vi "RD_WR_init.vi"(0 "MVIName def":string[](array[string]), 1 "N_moduls":i32, 2 "Status Reference":T2, 3 "KFM":string[](array[string]), 5 "IP addr def":T4(array[cluster]), 7 "timeouts def":T3[](array[typedef]), 9 "start_stop def":bool[](array[boolean]), 11 "error in":errorcluster, 12 "WR en def":bool[](array[boolean]), 13 "conninfo system DB":T1, 14 "KFMTable":string="kfm_3") -> (4 "RD_WR param":T5, 15 "error":errorcluster)   [LabVIEW 2019, in "ICPCON_Param.lvlib"]
uses:
  ICPCON_Param.lvlib
  ICPCON Param.ctl
  Eth timeouts.ctl
  Eth Status/Ctl/Status.ctl
  MB_TCP2/MB_TCP_State.ctl
  Database/ctl/Coninfo.ctl
  Eth Status/Eth Status.lvlib
  Database/PostgreSQL.lvlib
  MB_TCP2/MB_TCP.lvclass
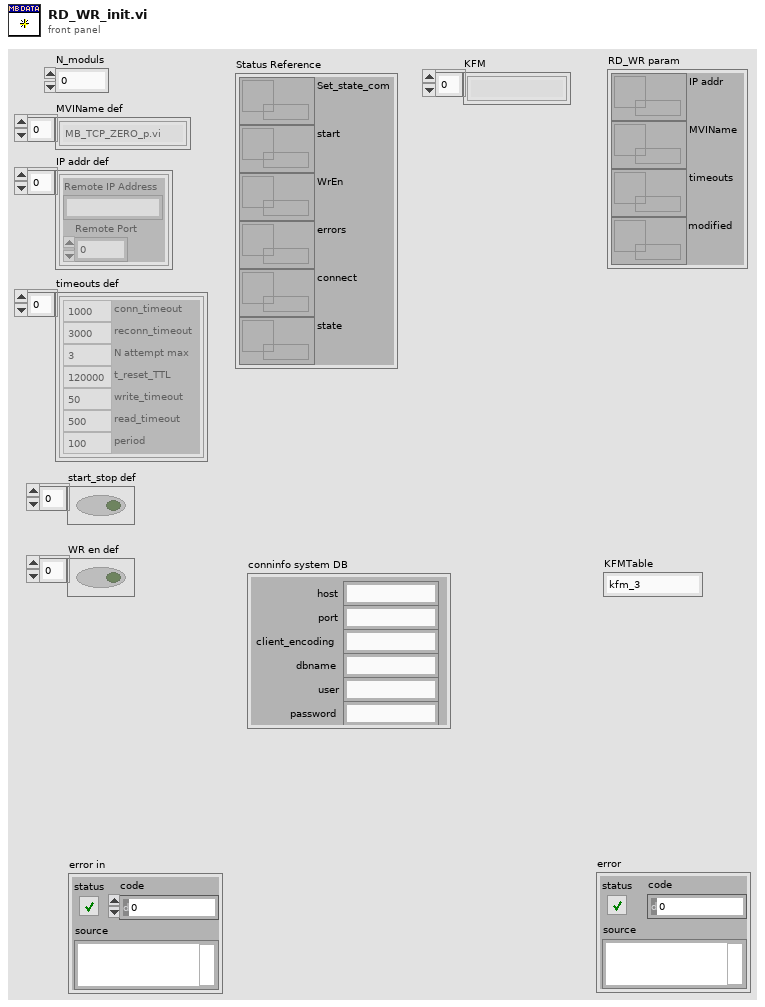
[diagram p1: front panel]
types:
  T1 = typedef "PostgreSQL.lvlib/Coninfo.ctl" = cluster{"host":string, "port":string, "client_encoding":string, "dbname":string, "user":string, "password":string}
  T2 = typedef "Eth Status.lvlib/Status.ctl" = cluster{"Set_state_com":refnum<data-value>, "start":refnum<data-value>, "WrEn":refnum<data-value>, "errors":refnum<data-value>, "connect":refnum<data-value>, "state":refnum<data-value>}
  T3 = typedef "ICPCON_Param.lvlib/Eth timeouts.ctl" = cluster{"conn_timeout":i32, "reconn_timeout":i32, "N attempt max":i32, "t_reset_TTL":i32, "write_timeout":i32, "read_timeout":i32, "period":i32}
  T4 = cluster{"Remote IP Address":string, "Remote Port":u16}[]
  T5 = typedef "ICPCON_Param.lvlib/ICPCON Param.ctl" = cluster{"IP addr":refnum<data-value>, "MVIName":refnum<data-value>, "timeouts":refnum<data-value>, "modified":refnum<data-value>}
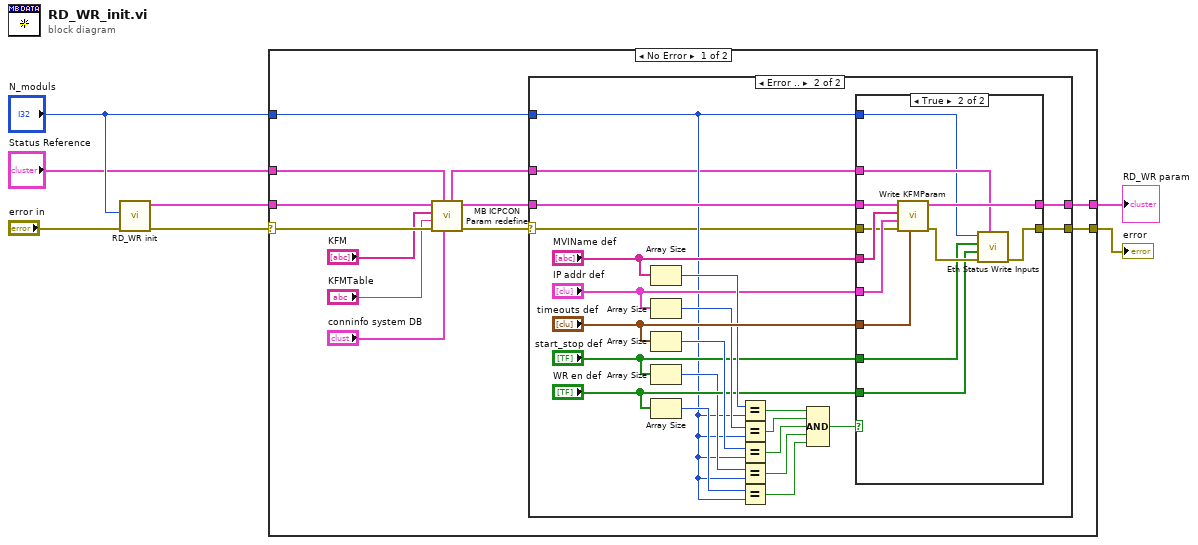
[diagram p0: block diagram]
diagram:
  n1 = call "RD_WR init.vi"("error in"="error in", "N_moduls"="N_moduls") -> ("error"=w2:errorcluster, "RD_WR param"=w5:T5)  [unwired: 8 in]
  n2 = case shown="No Error" w2 {
    selector: w2 -> [w14 w58]
    tunnel: [w18 w58] -> w3
    tunnel: w5 -> [w16 w59]
    tunnel: [w19 w59] -> w6
    tunnel: "N_moduls" -> [w15 _]
    tunnel: "Status Reference" -> [w13 _]
    frame No Error {
      n3 = call "MB ICPCON Param redefine.vi"("conninfo"="conninfo system DB", "Status Reference"=w13, "error in (no error)"=w14, "KFMTable"="KFMTable", "KFM param"="KFM", "KFM param in"=w16) -> ("error"=w11:errorcluster, "KFM param out"=w17:T5, "Status Reference out"=w12:T2)  [unwired: 3 in]
      n4 = case shown="Error .." w11 {
        selector: w11 -> [w20 w22]
        tunnel: [w20 w23] -> w18
        tunnel: w17 -> [w21 w43]
        tunnel: [w21 w25] -> w19
        tunnel: w15 -> [_ w26]
        tunnel: w12 -> [_ w24]
        frame No Error {
        }
        frame Error {
          n5 = Array Size(array="MVIName def") -> (size(s)=w39:i32)
          n6 = Array Size(array="IP addr def") -> (size(s)=w38:i32)
          n7 = Array Size(array="timeouts def") -> (size(s)=w37:i32)
          n8 = Array Size(array="start_stop def") -> (size(s)=w34:i32)
          n9 = Array Size(array="WR en def") -> (size(s)=w33:i32)
          n10 = Equal?(x=w39, y=w26) -> (x = y?=w40:bool)
          n11 = Equal?(x=w38, y=w26) -> (x = y?=w41:bool)
          n12 = Equal?(x=w37, y=w26) -> (x = y?=w32:bool)
          n13 = Equal?(x=w34, y=w26) -> (x = y?=w31:bool)
          n14 = Equal?(x=w33, y=w26) -> (x = y?=w30:bool)
          n15 = Compound Arithmetic op=AND(w40, w41, w32, w31, w30) -> (w29:bool)
          n16 = case shown="True" w29 {
            tunnel: "MVIName def" -> [_ w49]
            tunnel: "IP addr def" -> [_ w48]
            tunnel: [w44 w53] -> w23
            tunnel: w43 -> [w45 w57]
            tunnel: [w45 w56] -> w25
            tunnel: "timeouts def" -> [_ w55]
            tunnel: w24 -> [_ w52]
            tunnel: "start_stop def" -> [_ w51]
            tunnel: "WR en def" -> [_ w50]
            tunnel: w26 -> [_ w47]
            tunnel: w22 -> [w44 w46]
            frame False {
            }
            frame True {
              n17 = call "Write KFMParam.vi"("timeouts"=w55, "error in (no error)"=w46, "IP Address"=w48, "MVIName"=w49, "KFMParam in"=w57) -> ("error out"=w54:errorcluster, "KFMParam out"=w56:T5)  [unwired: 5 in]
              n18 = call "Eth Status Write Inputs.vi"("Status Reference"=w52, "error in (no error)"=w54, "Write Enable"=w50, "Start"=w51, "Lenght"=w47) -> ("error out"=w53:errorcluster)  [unwired: 5 in, 1 out]
            }
          }
        }
      }
    }
    frame Error {
    }
  }
  "error" <- w3
  "RD_WR param" <- w6
